vi "Barycentric Interpolation Method.vi"(10 "FFT array":dbl[](array[numeric])) -> (0 "max index(es)":i32, 3 "Index Bin":dbl)   [LabVIEW 2014]
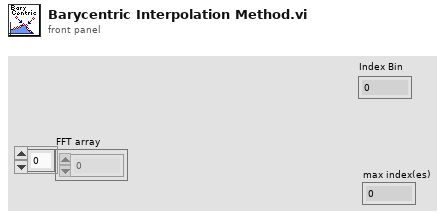
[diagram p1: front panel]
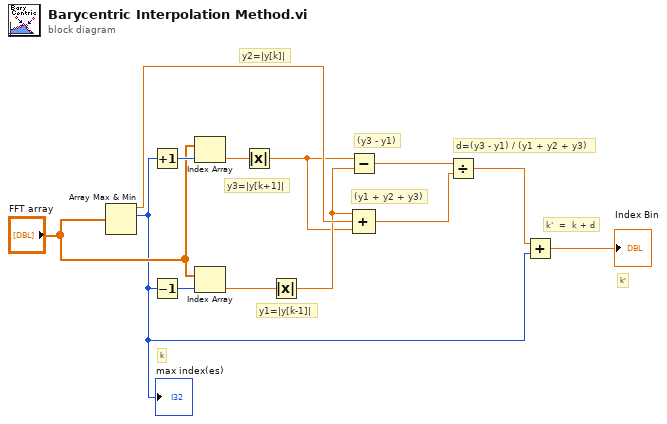
[diagram p0: block diagram]
diagram:
  # "k'"
  # "k'  =  k + d"
  # "d=(y3 - y1) / (y1 + y2 + y3)"
  # "(y1 + y2 + y3)"
  # "(y3 - y1)"
  # "y2=|y[k]|"
  # "k"
  # "y3=|y[k+1]|"
  # "y1=|y[k-1]|"
  n1 = Array Max & Min(array="FFT array") -> (max value=w8:dbl, max index (indices)=w2:i32)  [unwired: 2 out]
  "max index(es)" <- w2
  n2 = Increment(x=w2) -> (x+1=w12:i32)
  n3 = Decrement(x=w2) -> (x-1=w13:i32)
  n4 = Index Array(array="FFT array", index=w12) -> (element=w9:dbl)
  n5 = Index Array(array="FFT array", index=w13) -> (element=w10:dbl)
  n6 = Absolute Value(x=w9) -> (abs(x)=w6:dbl)
  n7 = Absolute Value(x=w10) -> (abs(x)=w7:dbl)
  n8 = Subtract(x=w6, y=w7) -> (x-y=w5:dbl)
  n9 = Compound Arithmetic op=ADD(w7, w8, w6) -> (w4:dbl)
  n10 = Divide(x=w5, y=w4) -> (x/y=w3:dbl)
  n11 = Add(x=w3, y=w2) -> (x+y=→"Index Bin":dbl)
